vi "niDTS Template RF Test Get Default Limits.vi"(0 "Template Tx Test Handle in":T2, 11 "error in (no error)":errorcluster) -> (4 "Template Tx Test Handle out":T2, 6 "USL":T1, 8 "LSL":T1, 15 "error out":errorcluster)   [LabVIEW 2014, in "niDTS Template.lvlib"]
uses:
  niDTS Template.lvlib
  Includes/Template RF Test INC Handle.ctl
  Objects/BASE_class/Template RF Test.lvclass
  Includes/Template RF Test INC Results.ctl
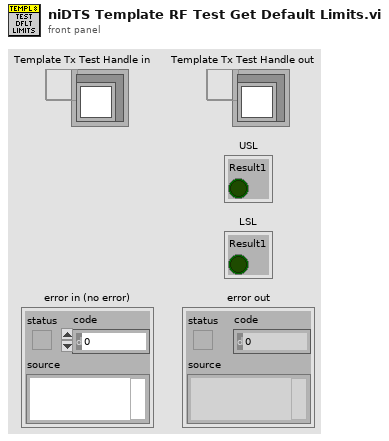
[diagram p1: front panel]
types:
  T1 = typedef "niDTS Template.lvlib/Template RF Test INC Results.ctl" = cluster{"Result1":bool}
  T2 = typedef "niDTS Template.lvlib/Template RF Test INC Handle.ctl" = refnum<data-value>
  T3 = typedef "Template.lvlib/Template Tx Test INC Results.ctl" = cluster{"Result1":bool}
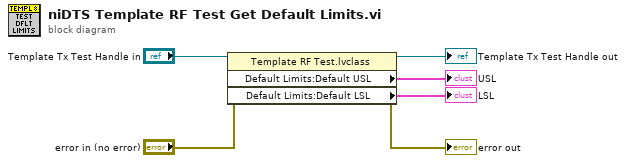
[diagram p0: block diagram]
diagram:
  n1 = property class="Template RF Test.lvclass"(reference="Template Tx Test Handle in", error in="error in (no error)") -> (reference out=→"Template Tx Test Handle out":T2, error out=→"error out":errorcluster, "Default Limits:Default USL"=→"USL":T3, "Default Limits:Default LSL"=→"LSL":T3)
